vi "Read DurationTicks.vi"(8 "error in (no error)":errorcluster, 11 "State in":refnum<class "State.lvclass">) -> (0 "error out":errorcluster, 2 "DurationTicks":u32, 3 "State out":refnum<class "State.lvclass">)   [LabVIEW 2013, in "State.lvclass"]
uses:
  State.lvclass
  State.lvclass/State.ctl
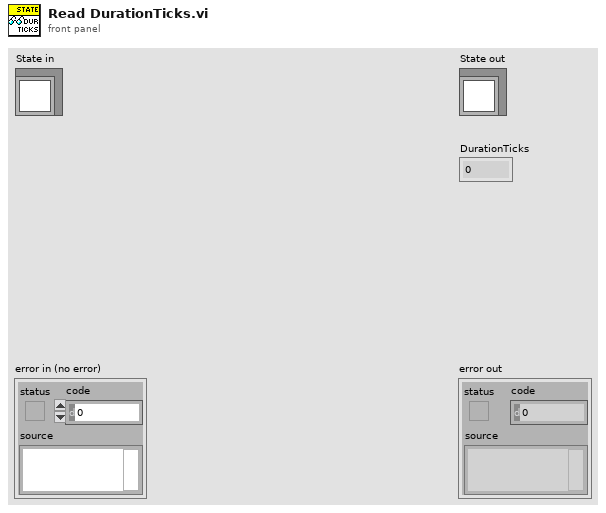
[diagram p1: front panel]
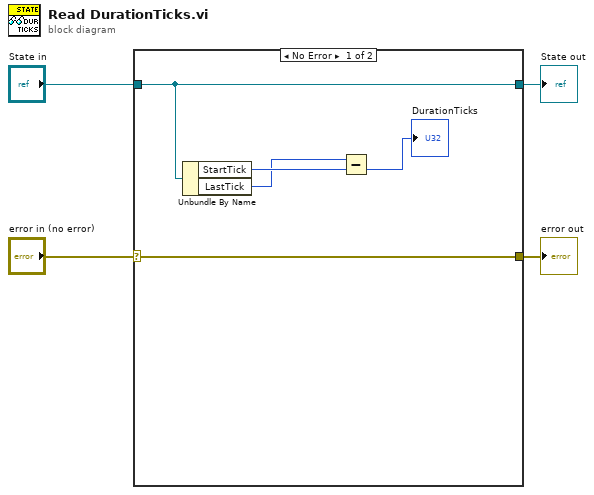
[diagram p0: block diagram]
diagram:
  n1 = case shown="No Error" "error in (no error)" {
    selector: "error in (no error)" -> [w9 w10]
    tunnel: [w9 w10] -> w3
    tunnel: [w8 w11] -> w1
    tunnel: "State in" -> [w8 w11]
    frame No Error {
      n2 = Unbundle By Name(w8) -> ("StartTick"=w7:u32, "LastTick"=w5:u32)
      n3 = Subtract(x=w5, y=w7) -> (x-y=→"DurationTicks":u32)
    }
    frame Error {
    }
  }
  "error out" <- w3
  "State out" <- w1
